vi "Codigo para buscar.vi"() -> ()   [LabVIEW 2020]
panel:
  out "x .and. y? 4":bool
  in  "x 4":bool
  in  "y 4":bool
  out "appended array":dbl[](array[numeric])
  in  "element":dbl
  out "x .and. y? 3":bool
  in  "x 3":bool
  in  "y 3":bool
  out "x .and. y? 2":bool
  in  "x 2":bool
  in  "y 2":bool
  out "x .and. y?":bool
  in  "x":bool
  in  "y":bool
  out "Waveform Chart":dbl(graph)
  out "String":string
  in  "Numeric":dbl
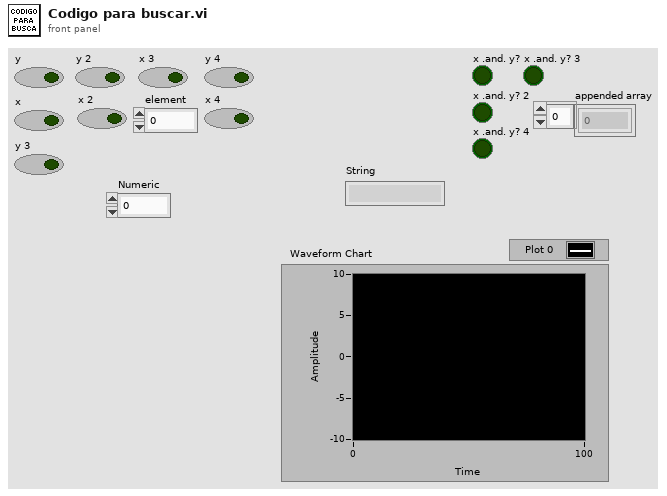
[diagram p1: front panel]
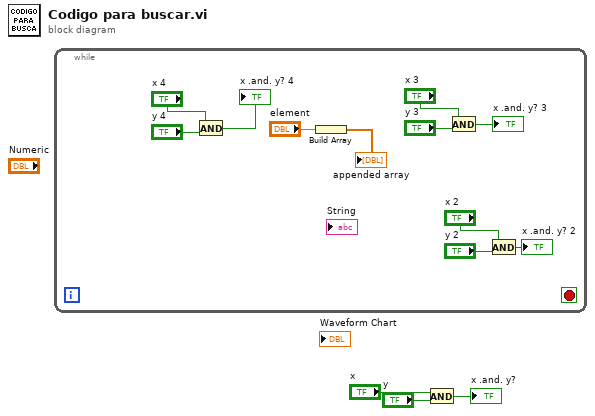
[diagram p0: block diagram]
diagram:
  n1 = while {
    stop <- _ stop-if-true
    n2 = And(x="x 4", y="y 4") -> (x .and. y?=→"x .and. y? 4":bool)
    n3 = Build Array("element") -> (→"appended array":dbl[])
    n4 = And(x="x 3", y="y 3") -> (x .and. y?=→"x .and. y? 3":bool)
    n5 = And(x="x 2", y="y 2") -> (x .and. y?=→"x .and. y? 2":bool)
  }
  n6 = And(x="x", y="y") -> (x .and. y?=→"x .and. y?":bool)
